vi "Waveform Capture.vi"(8 "error in (no error)":errorcluster, 11 "AirSAS Controls":T1={"Receive Duration"=0.0, "I/O"={"DAQmx Device"="Dev1", "AO Range"=0.0, "AI Range"=0.0, "DAQ Group Delay"=0.0, "Fs"=0.0}, "Hardware"={"Centerpos"=[0.0, 0.0, 0.0], "TXpos"=[0.0, 0.0, 0.0], "RX1pos"=[0.0, 0.0, 0.0], "RX2pos"=[0.0, 0.0, 0.0], "Angle"=0.0, "Height"=0.0}, "Waveform"={"LFM Parameters"={"Duration"=1.0, "Fstart (Hz)"=1000.0, "Fstop (Hz)"=10000.0, "Out. Amplitude (Vpk)"=1.0, "Window %"=10.0}, "Transmit Waveform"={"t0"=timestamp(0 s since 1904-01-01), "dt"=1.0, "Y"=[]}}, "LINX Resource"={"IO"=enum."Remote", "Interface"=enum."Serial", "LINX Device Config"={"Interface"=enum."Serial", "COM Port"="COM13", "TCP Configuration"={"IP Address"="", "Port"=0}, "Device Family"=1, "Device ID"=1, "Device Name"="myRIO-1900", "TCP Ref"=refnum, "Channels"={"DI"=[0, 1, 2, 3, 4, 5, 6, 7, 8, 9, 10, 11, 12, 13, 14, 15, 16, 17, 18, 19, 20, 21, 22, 23, 24, 25, 26, 27, 28, 29, 30, 31, 32, 33, 34, 35, 36, 37, 38, 39, 40, 41, 42, 43, 44, 45, 46], "DO"=[0, 1, 2, 3, 4, 5, 6, 7, 8, 9, 10, 11, 12, 13, 14, 15, 16, 17, 18, 19, 20, 21, 22, 23, 24, 25, 26, 27, 28, 29, 30, 31, 32, 33, 34, 35, 36, 37, 38, 39, 40, 41, 42, 43, 44, 45, 46], "AI"=[0, 1, 2, 3, 4, 5, 6, 7, 8, 9, 10, 11], "AO"=[], "PWM"=[3, 5, 6, 9, 10], "QE"=[], "UART"=[0, 1], "I2C 2"=[0], "SPI"=[0], "CAN"=[], "Servo"=[], "AI Ref (V)"=0.0, "AI Resolution (Bits)"=0, "AO Ref (V)"=0.0, "AO Resolution (Bits)"=0}}}, "Port"=3000.0} {"Waveform"."LFM Parameters"."Window %" format="%.2g"; "Waveform"."LFM Parameters"."Out. Amplitude (Vpk)" format="%0.2f"; "Waveform"."LFM Parameters"."Fstop (Hz)" format="%^.3e"; "Waveform"."LFM Parameters"."Fstart (Hz)" format="%^.3e"; "Waveform"."LFM Parameters"."Duration" format="%.3f"}) -> (0 "error in (no error) 2":errorcluster, 3 "AirSAS Controls 2":T1={"Receive Duration"=0.0, "I/O"={"DAQmx Device"="Dev1", "AO Range"=0.0, "AI Range"=0.0, "DAQ Group Delay"=0.0, "Fs"=0.0}, "Hardware"={"Centerpos"=[0.0, 0.0, 0.0], "TXpos"=[0.0, 0.0, 0.0], "RX1pos"=[0.0, 0.0, 0.0], "RX2pos"=[0.0, 0.0, 0.0], "Angle"=0.0, "Height"=0.0}, "Waveform"={"LFM Parameters"={"Duration"=1.0, "Fstart (Hz)"=1000.0, "Fstop (Hz)"=10000.0, "Out. Amplitude (Vpk)"=1.0, "Window %"=10.0}, "Transmit Waveform"={"t0"=timestamp(0 s since 1904-01-01), "dt"=1.0, "Y"=[]}}, "LINX Resource"={"IO"=enum."Remote", "Interface"=enum."Serial", "LINX Device Config"={"Interface"=enum."Serial", "COM Port"="COM13", "TCP Configuration"={"IP Address"="", "Port"=0}, "Device Family"=1, "Device ID"=1, "Device Name"="myRIO-1900", "TCP Ref"=refnum, "Channels"={"DI"=[0, 1, 2, 3, 4, 5, 6, 7, 8, 9, 10, 11, 12, 13, 14, 15, 16, 17, 18, 19, 20, 21, 22, 23, 24, 25, 26, 27, 28, 29, 30, 31, 32, 33, 34, 35, 36, 37, 38, 39, 40, 41, 42, 43, 44, 45, 46], "DO"=[0, 1, 2, 3, 4, 5, 6, 7, 8, 9, 10, 11, 12, 13, 14, 15, 16, 17, 18, 19, 20, 21, 22, 23, 24, 25, 26, 27, 28, 29, 30, 31, 32, 33, 34, 35, 36, 37, 38, 39, 40, 41, 42, 43, 44, 45, 46], "AI"=[0, 1, 2, 3, 4, 5, 6, 7, 8, 9, 10, 11], "AO"=[], "PWM"=[3, 5, 6, 9, 10], "QE"=[], "UART"=[0, 1], "I2C 2"=[0], "SPI"=[0], "CAN"=[], "Servo"=[], "AI Ref (V)"=0.0, "AI Resolution (Bits)"=0, "AO Ref (V)"=0.0, "AO Resolution (Bits)"=0}}}, "Port"=3000.0} {"Waveform"."LFM Parameters"."Window %" format="%.2g"; "Waveform"."LFM Parameters"."Out. Amplitude (Vpk)" format="%0.2f"; "Waveform"."LFM Parameters"."Fstop (Hz)" format="%^.3e"; "Waveform"."LFM Parameters"."Fstart (Hz)" format="%^.3e"; "Waveform"."LFM Parameters"."Duration" format="%.3f"})   [LabVIEW 2021]
uses:
  controls/Air SAS Controls.ctl
  <vilib>/MakerHub/LINX/Private/Type Defs/LINX Ref.ctl
  <vilib>/MakerHub/LINX/Private/Type Defs/Platform.ctl
  <vilib>/MakerHub/LINX/Private/Type Defs/Interface.ctl
  <vilib>/MakerHub/LINX/Private/Device/Type Defs/LINX Device Config.ctl
  <vilib>/MakerHub/LINX/Private/Device/Type Defs/TCP Config.ctl
  <vilib>/MakerHub/LINX/Private/Device/Type Defs/Channels.ctl
  <vilib>/Analysis/4window.llb/Cosine Tapered Window (DBL).vi
  <vilib>/Utility/file.llb/Write Delimited Spreadsheet (DBL).vi
  <vilib>/Analysis/NI_AALBase.lvlib
  <vilib>/Analysis/NI_AALPro.lvlib
  <vilib>/MakerHub/LINX/LMH-LINX.lvlib
  <vilib>/MakerHub/LINX/Private/Device/Device.lvlib
panel:
  in  "Interpulse Delay":dbl=1.0 caption="Delay Time (s)"
  out "Captured Data":waveform(dbl)(graph)
  in  "Receive Duration":dbl=0.01
  in  "Waveform Name":string
  in  "base path":path
  out "Analytic Waveform":waveform(dbl)(graph)
  in  "Start Capture":bool
  in  "Number of Captures":i32=10
  in  "stop":bool
  in  "Gen Wfm":bool
  in  "LFM Parameters":T8={"Fs (Hz)"=100000.0, "Sweep Length (s)"=0.001, "Fstart (Hz)"=10000.0, "Fstop (Hz)"=10000.0, "Out. Amplitude (Vpk)"=1.0, "Window %"=10.0} {"Window %" format="%.2g"; "Out. Amplitude (Vpk)" format="%0.2f"; "Fstop (Hz)" format="%^.3e"; "Fstart (Hz)" format="%^.3e"; "Sweep Length (s)" format="%.3f"; "Fs (Hz)" min=1000.0 max=2000000.0 format="%^.0e"}
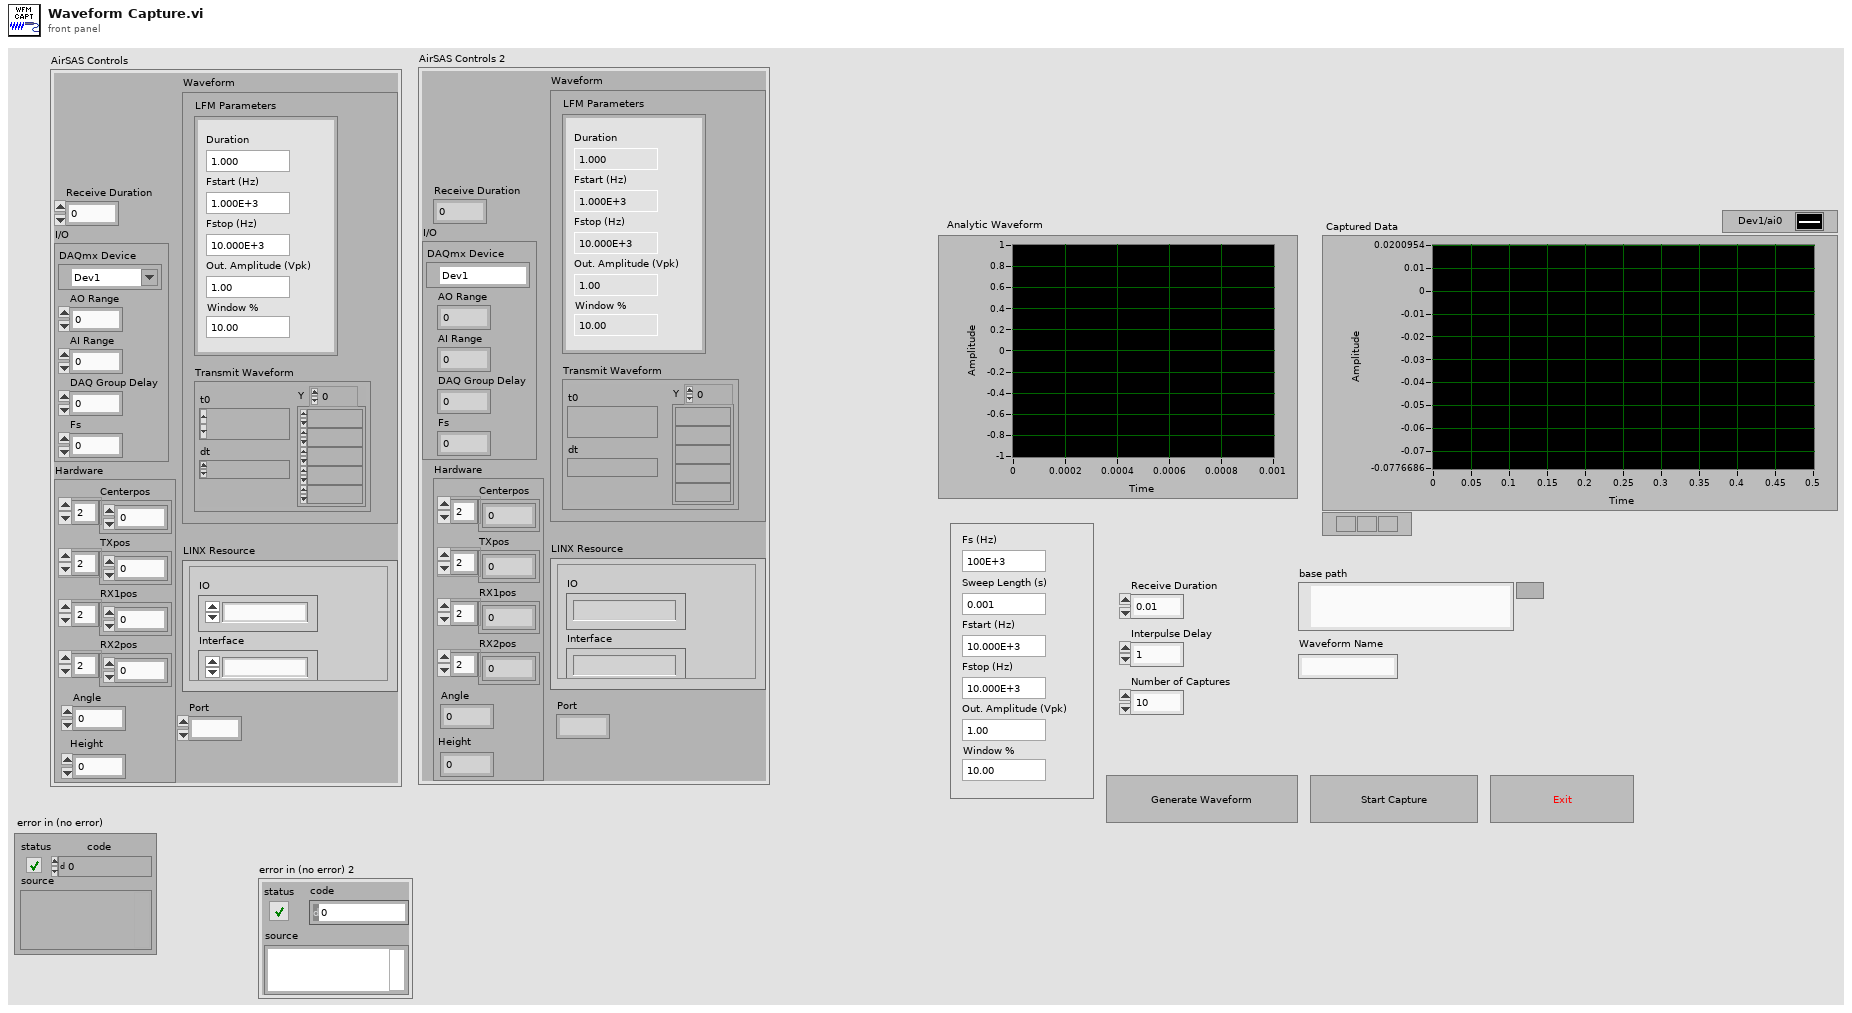
[diagram p1: front panel]
types:
  T1 = typedef "Air SAS Controls.ctl" = cluster{"Receive Duration":dbl, "I/O":cluster{"DAQmx Device":tag, "AO Range":dbl, "AI Range":dbl, "DAQ Group Delay":dbl, "Fs":dbl}, "Hardware":cluster{"Centerpos":dbl[], "TXpos":dbl[], "RX1pos":dbl[], "RX2pos":dbl[], "Angle":dbl, "Height":dbl}, "Waveform":cluster{"LFM Parameters":cluster{"Duration":dbl, "Fstart (Hz)":dbl, "Fstop (Hz)":dbl, "Out. Amplitude (Vpk)":dbl, "Window %":dbl}, "Transmit Waveform":waveform(dbl)}, "LINX Resource":T2, "Port":dbl}
  T2 = typedef "LMH-LINX.lvlib/LINX Ref.ctl" = cluster{"IO":T3, "Interface":T4, "LINX Device Config":T5}
  T3 = typedef "LMH-LINX.lvlib/Platform.ctl" = enum16{"Remote", "Local"}
  T4 = typedef "LMH-LINX.lvlib/Interface.ctl" = enum16{"Serial", "TCP"}
  T5 = typedef "LMH-LINX.lvlib/Device.lvlib/LINX Device Config.ctl" = cluster{"Interface":T4, "COM Port":refnum<visa-resource-name>, "TCP Configuration":T6, "Device Family":u8, "Device ID":u8, "Device Name":string, "TCP Ref":refnum<k5>, "Channels":T7}
  T6 = typedef "LMH-LINX.lvlib/Device.lvlib/TCP Config.ctl" = cluster{"IP Address":string, "Port":u16}
  T7 = typedef "LMH-LINX.lvlib/Channels.ctl" = cluster{"DI":u8[], "DO":u8[], "AI":u8[], "AO":u8[], "PWM":u8[], "QE":u8[], "UART":u8[], "I2C 2":u8[], "SPI":u8[], "CAN":u8[], "Servo":u8[], "AI Ref (V)":dbl, "AI Resolution (Bits)":u8, "AO Ref (V)":dbl, "AO Resolution (Bits)":u8}
  T8 = cluster{"Fs (Hz)":dbl, "Sweep Length (s)":dbl, "Fstart (Hz)":dbl, "Fstop (Hz)":dbl, "Out. Amplitude (Vpk)":dbl, "Window %":dbl}
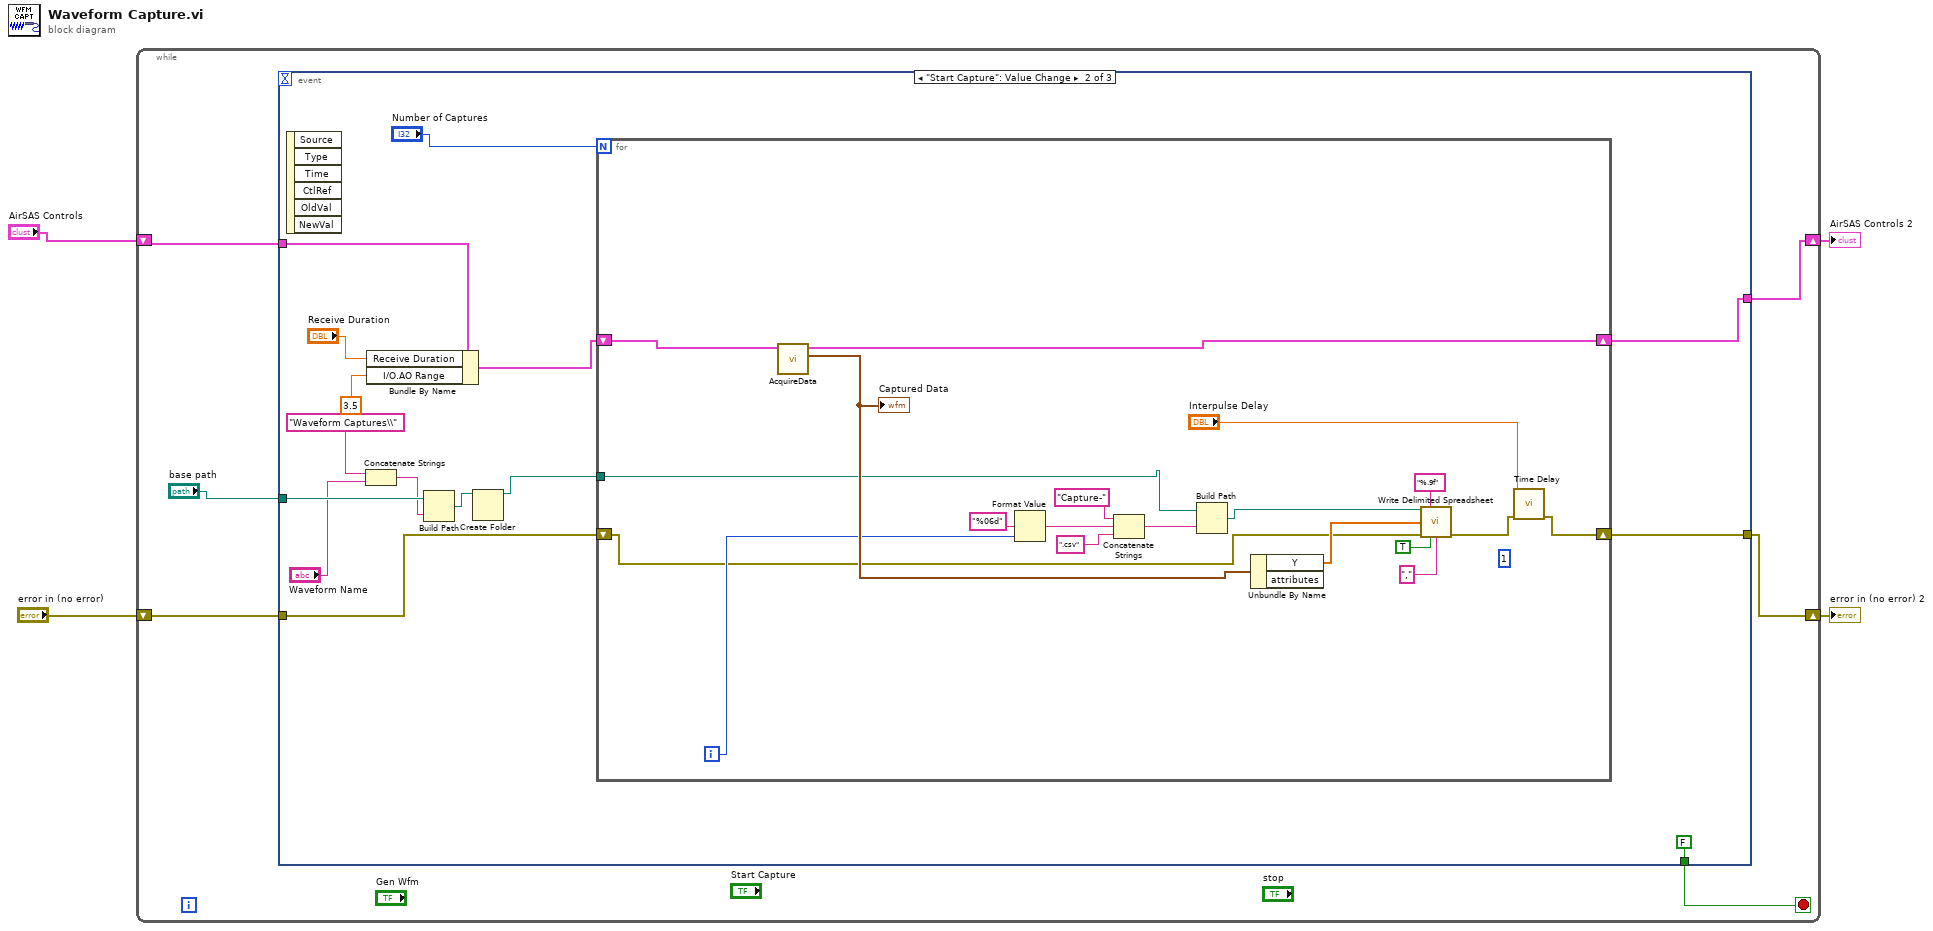
[diagram p0: block diagram]
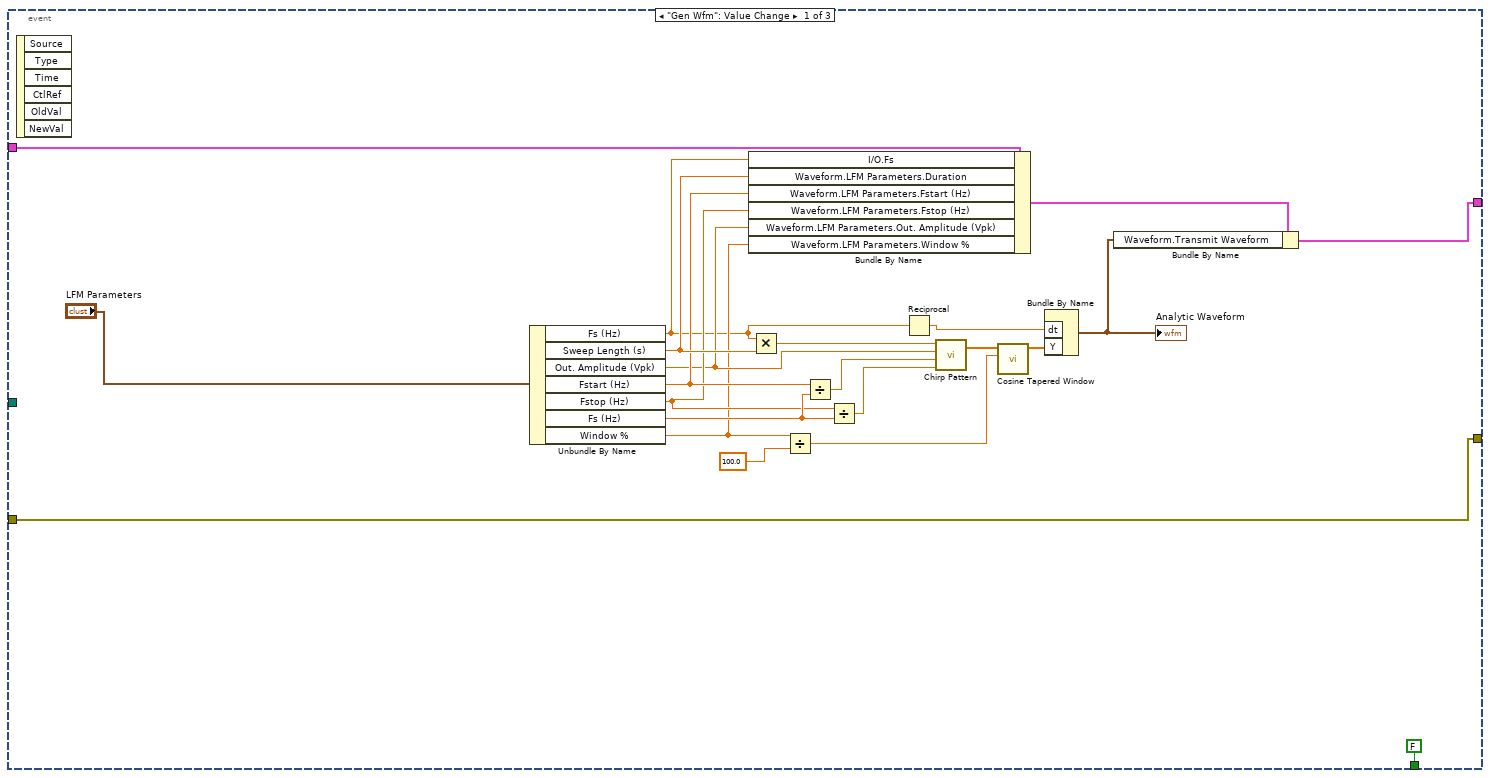
[diagram p2: hidden frame]
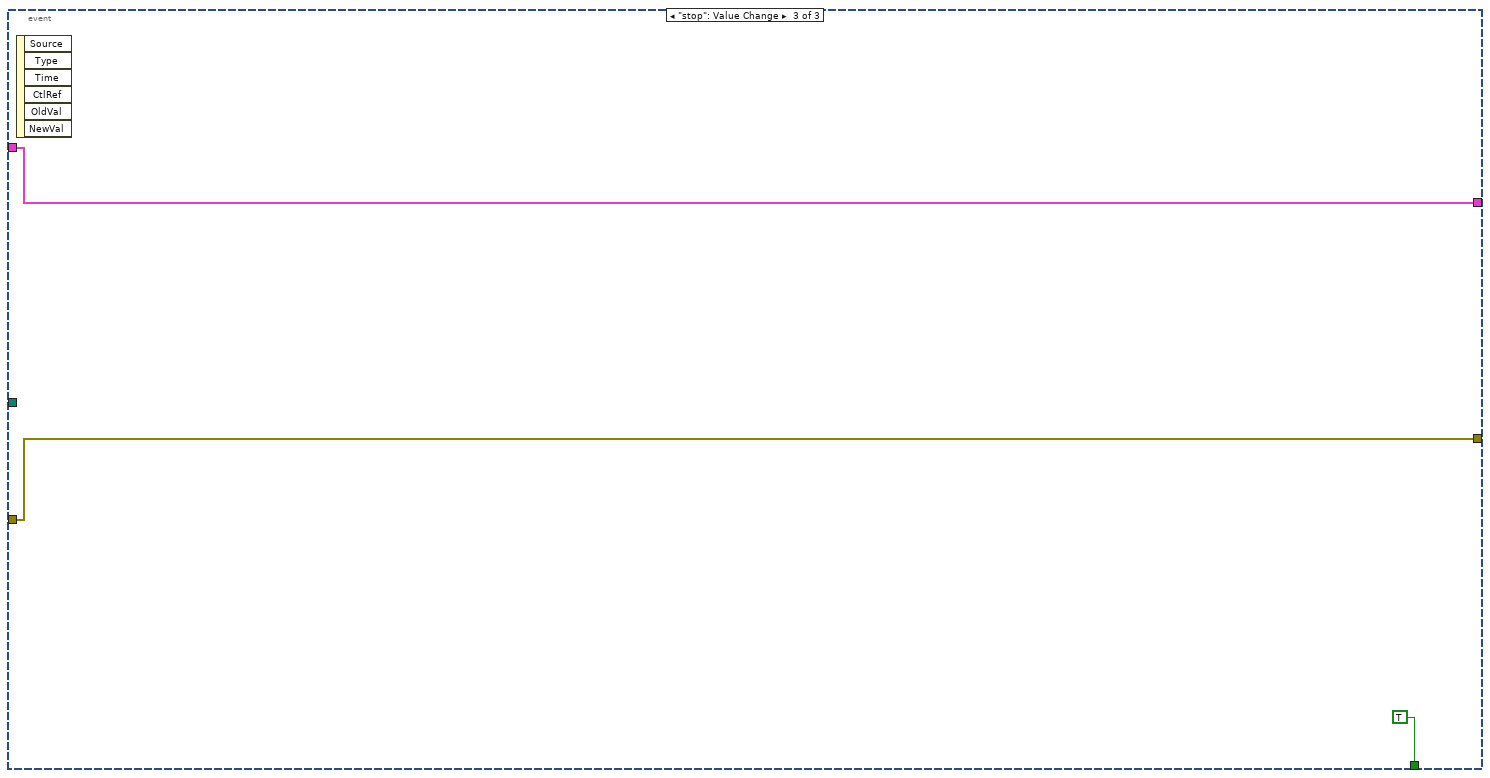
[diagram p3: hidden frame]
diagram:
  n1 = while {
    shift-right: [w8] -> w3
    shift-left: "AirSAS Controls" -> [w9]
    shift-right: [w6] -> w1
    shift-left: "error in (no error)" -> [w5]
    stop <- w10 stop-if-true
    n2 = event shown="[1] \"Start Capture\": Value Change" {
      selector: _ -> [_ _ _]
      dyn-events: _ -> [_ _ _]
      timeout: _ -> [_ _ _]
      tunnel: [FALSE FALSE TRUE] -> w10
      tunnel: w9 -> [w14 w35 w67]
      tunnel: [w11 w46 w67] -> w8
      tunnel: "base path" -> [_ w44 _]
      tunnel: [w13 w39 w68] -> w6
      tunnel: w5 -> [w13 w38 w68]
      event "Gen Wfm": Value Change {
        n3 = event-data() -> ()  [unwired: 1 in, 6 out]
        n4 = Unbundle By Name("LFM Parameters") -> ("Fs (Hz)"=w16:dbl, "Sweep Length (s)"=w22:dbl, "Out. Amplitude (Vpk)"=w19:dbl, "Fstart (Hz)"=w21:dbl, "Fstop (Hz)"=w20:dbl, "Fs (Hz)"=w29:dbl, "Window %"=w18:dbl)
        n5 = Bundle By Name(cluster=w14, "I/O.Fs"=w16, "Waveform.LFM Parameters.Duration"=w22, "Waveform.LFM Parameters.Fstart (Hz)"=w21, "Waveform.LFM Parameters.Fstop (Hz)"=w20, "Waveform.LFM Parameters.Out. Amplitude (Vpk)"=w19, "Waveform.LFM Parameters.Window %"=w18) -> (w12:T1)
        n6 = Multiply(x=w16, y=w22) -> (x*y=w31:dbl)
        n7 = Divide(x=w18, y=100.0) -> (x/y=w24:dbl)
        n8 = Divide(x=w21, y=w29) -> (x/y=w30:dbl)
        n9 = Divide(x=w20, y=w29) -> (x/y=w28:dbl)
        n10 = Reciprocal(x=w16) -> (1/x=w25:dbl)
        n11 = call <vilib>:"Chirp Pattern.vi"("f2"=w28, "f1"=w30, "amplitude"=w19, "samples"=w31) -> ("Chirp Pattern"=w27:dbl[])  [unwired: 1 out]
        n12 = call-poly <vilib>:"Cosine Tapered Window.vi"("ratio"=w24, "X"=w27) -> ("Windowed X"=w26:dbl[])  [unwired: 8 in, 1 out]
        n13 = Bundle By Name("dt"=w25, "Y"=w26) -> (w17:waveform(dbl))  [unwired: 1 in]
        "Analytic Waveform" <- w17
        n14 = Bundle By Name(cluster=w12, "Waveform.Transmit Waveform"=w17) -> (w11:T1)
      }
      event "Start Capture": Value Change {
        n15 = event-data() -> ()  [unwired: 1 in, 6 out]
        n16 = Concatenate Strings("Waveform Captures\\" ("time format string (%c)"), "Waveform Name") -> (w41:string)
        n17 = Bundle By Name(cluster=w35, "Receive Duration"="Receive Duration", "I/O.AO Range"=3.5) -> (w34:T1)
        n18 = Build Path(base path=w44, name or relative path=w41) -> (appended path=w45:path)
        n19 = Create Folder(path (use dialog)=w45) -> (created path=w40:path)  [unwired: 2 in, 2 out]
        n20 = for {
          N: "Number of Captures" -> [_]
          shift-right: [w65] -> w46
          shift-left: w34 -> [w66]
          tunnel: w40 -> [w52]
          shift-right: [w48] -> w39
          shift-left: w38 -> [w51]
          i -> [w53]
          (unwired) 1 ("y")
          n21 = call "AcquireData.vi"("AirSAS Controls In"=w66) -> ("data"=w54:waveform(dbl), "AirSAS Controls Out"=w65:T1)  [unwired: 8 in, 1 out]
          "Captured Data" <- w54
          n22 = Format Value(format string="%06d", value (0)=w53) -> (output string=w61:string)  [unwired: 1 in]
          n23 = Concatenate Strings("Capture-" ("string"), w61, ".csv") -> (w64:string)
          n24 = Build Path(base path=w52, name or relative path=w64) -> (appended path=w58:path)
          n25 = Unbundle By Name(w54) -> ("Y"=w59:dbl[])  [unwired: 1 out]
          n26 = call-poly <vilib>:"Write Delimited Spreadsheet.vi"("file path (dialog if empty)"=w58, "format (%.3f)"="%.9f" ("format string"), "1D data"=w59, "error in (no error)"=w51, "transpose? (no:F)"=TRUE, "delimiter (\\t)"="," ("delimiter (Tab)")) -> ("error out"=w49:errorcluster)  [unwired: 8 in, 1 out]
          n27 = call "Time Delay"("error in (no error)"=w49, "Delay Time (s)"="Interpulse Delay") -> ("error out"=w48:errorcluster)  [unwired: 9 in]
        }
      }
      event "stop": Value Change {
        n28 = event-data() -> ()  [unwired: 1 in, 6 out]
      }
    }
  }
  "AirSAS Controls 2" <- w3
  "error in (no error) 2" <- w1
